vi "DIM_Reset.vi"(8 "error in (no error)":errorcluster, 11 "UI_Actor in":refnum<class "UI_Actor.lvclass">) -> (0 "error out":errorcluster, 3 "UI_Actor out":refnum<class "UI_Actor.lvclass">)   [LabVIEW 2020, in "UI_Actor.lvlib" / "UI_Actor.lvclass"]
uses:
  UI_Actor.lvclass
  UI_Actor.lvclass/UI_Actor.ctl
  ctl_InternalMapItem.ctl
  support/Databox.lvlibp/TypesTools/Config/Config.lvclass
  support/Databox.lvlibp/TypesTools/Data/Data.lvclass
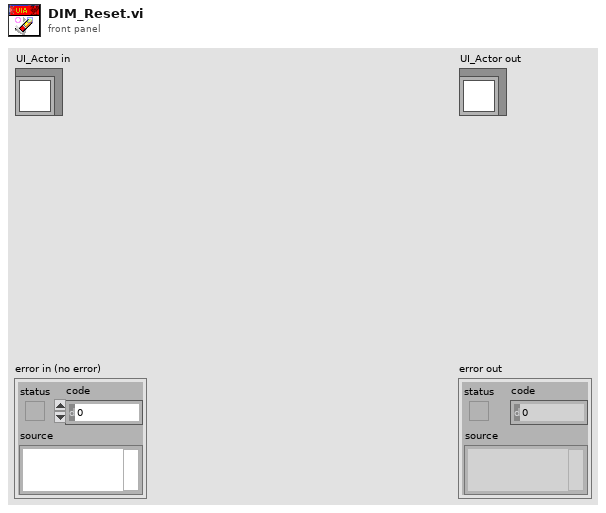
[diagram p1: front panel]
types:
  T1 = typedef "UI_Actor.lvlib/UI_Actor.lvclass/ctl_InternalMapItem.ctl" = cluster{"Config":refnum<class "Config.lvclass">, "LatestData":refnum<class "Data.lvclass">}
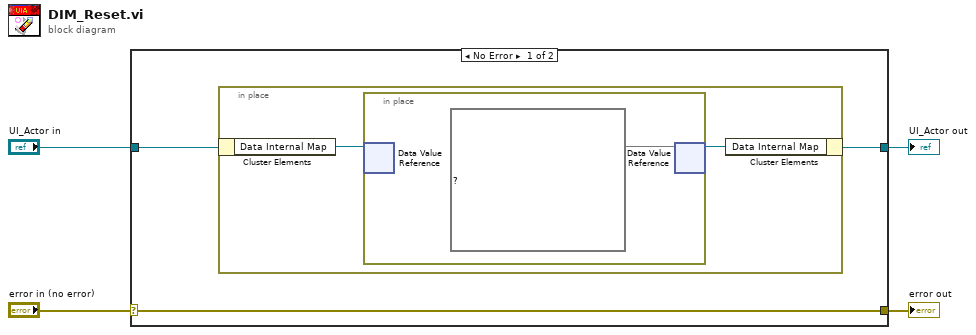
[diagram p0: block diagram]
diagram:
  n1 = case shown="No Error" "error in (no error)" {
    selector: "error in (no error)" -> [w7 w12]
    tunnel: [w7 w12] -> w3
    tunnel: [w5 w11] -> w1
    tunnel: "UI_Actor in" -> [w6 w11]
    frame No Error {
      n2 = in-place {
        n3 = in-place-cluster #1(w6) -> ("Data Internal Map"=w9:refnum<data-value>)
        n4 = in-place {
          n5 = in-place-dvr #2(w9) -> ()  [unwired: 2 out]
          n6 = in-place-dvr #2(map{string, map{string, T1}} {} ("data value")) -> (w8:refnum<data-value>)  [unwired: 1 out]
        }
        n7 = in-place-cluster #1("Data Internal Map"=w8) -> (w5:refnum<class "UI_Actor.lvclass">)
      }
    }
    frame Error {
    }
  }
  "error out" <- w3
  "UI_Actor out" <- w1
